vi "Write Numeric Type.vi"(8 "error in (no error)":errorcluster, 10 "Numeric Type":T1=enum."I32", 11 "Number Writer in":refnum<class "Number Writer.lvclass">) -> (0 "error out":errorcluster, 3 "Number Writer out":refnum<class "Number Writer.lvclass">)   [LabVIEW 2013, in "Number Writer.lvclass"]
doc: "Copyright (c) 2016 Sze Howe Koh\n\nThis Source Code Form is subject to the terms of the Mozilla Public License, v. 2.0. If a copy of the MPL was not distributed with this file, You can obtain one at http://mozilla.org/MPL/2.0/."
uses:
  Number Writer.lvclass
  Numeric Type.ctl
  Number Writer.lvclass/Number Writer.ctl
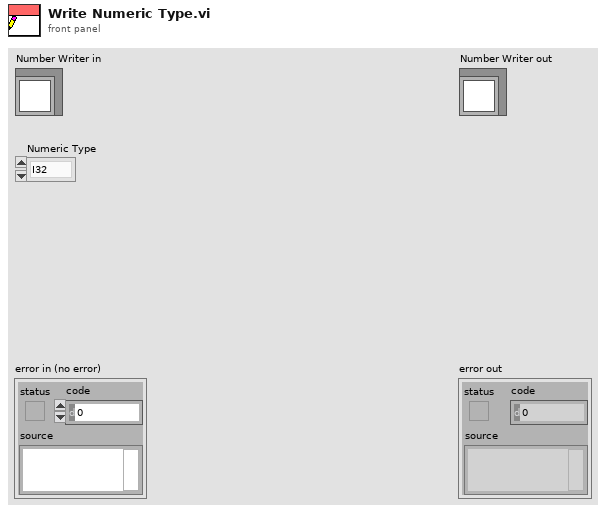
[diagram p1: front panel]
types:
  T1 = typedef "Number Writer.lvclass/Numeric Type.ctl" = enum16{"I8", "I16", "I32", "I64", "U8", "U16", "U32", "U64", "SGL", "DBL", "PTR INT", "PTR UINT"}
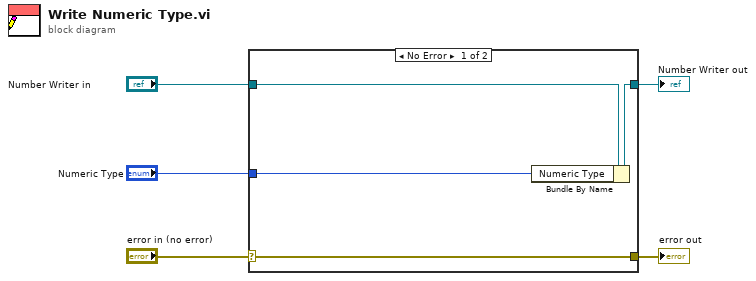
[diagram p0: block diagram]
diagram:
  n1 = case shown="No Error" "error in (no error)" {
    selector: "error in (no error)" -> [w9 w10]
    tunnel: [w9 w10] -> w4
    tunnel: [w7 w11] -> w2
    tunnel: "Number Writer in" -> [w8 w11]
    tunnel: "Numeric Type" -> [w6 _]
    frame No Error {
      n2 = Bundle By Name(cluster=w8, "Numeric Type"=w6) -> (w7:refnum<class "Number Writer.lvclass">)
    }
    frame Error {
    }
  }
  "error out" <- w4
  "Number Writer out" <- w2
